vi "TestStand.DisplayError.vi"(8 "error in (no error)":errorcluster, 11 "Application Manager":refnum<k7>) -> (0 "error out":errorcluster)   [LabVIEW 2015, in "Main.GUI.lvlib"]
doc: "This VI displays an error dialog in the event of an error."
uses:
  Main.GUI.lvlib
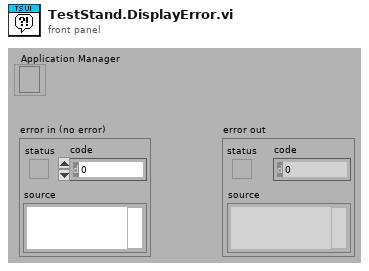
[diagram p1: front panel]
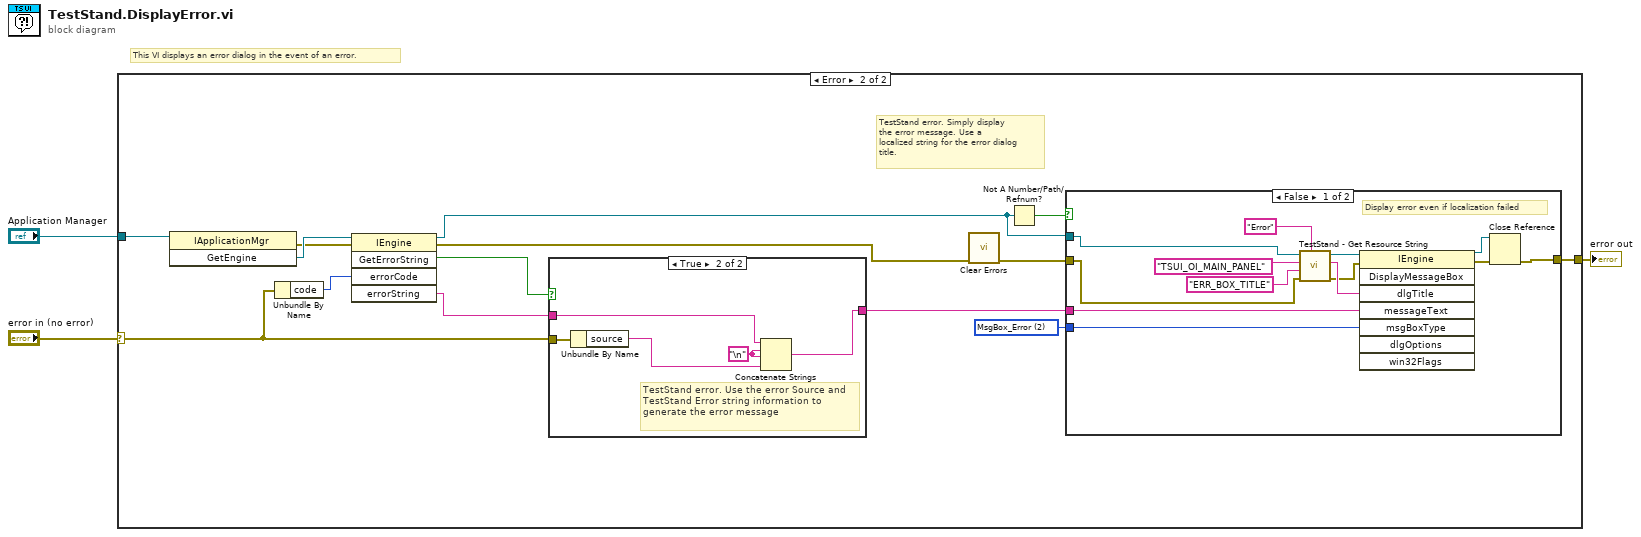
[diagram p0: block diagram]
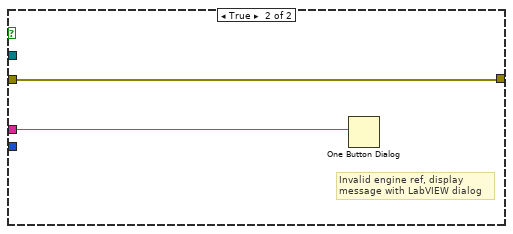
[diagram p3: hidden frame]
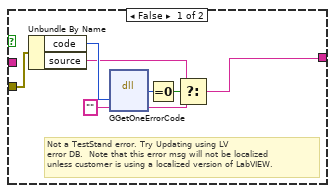
[diagram p4: hidden frame]
diagram:
  # "This VI displays an error dialog in the event of an error."
  n1 = case shown="Error" "error in (no error)" {
    selector: "error in (no error)" -> [w4 w16]
    tunnel: [w4 w12] -> w2
    tunnel: "Application Manager" -> [_ w13]
    frame No Error {
    }
    frame Error {
      w10 = 2 items=["MsgBox_Warning", "MsgBox_Information", "MsgBox_Error", "MsgBox_Custom"] ("msgBoxType")
      # "TestStand error. Simply display\nthe error message. Use a\nlocalized string for the error dialog\ntitle."
      n2 = invoke class="IApplicationMgr" method="GetEngine"(reference=w13) -> (error out=w14:errorcluster, "GetEngine"=w15:refnum<k7>)  [unwired: 2 in, 1 out]
      n3 = Unbundle By Name(w16) -> ("code"=w18:i32)
      n4 = invoke class="IEngine" method="GetErrorString"(reference=w15, error in=w14, "errorCode"=w18) -> (reference out=w5:refnum<k7>, error out=w6:errorcluster, "GetErrorString"=w17:bool, "errorString"=w8:string)  [unwired: 2 in, 1 out]
      n5 = case shown="True" w17 {
        tunnel: w16 -> [w35 w43]
        tunnel: [w34 w45] -> w11
        tunnel: w8 -> [_ w44]
        frame False {
          # "Not a TestStand error. Try Updating using LV\nerror DB.  Note that this error msg will not be localized\nunless customer is using a localized version of LabVIEW."
          n6 = Unbundle By Name(w35) -> ("code"=w37:i32, "source"=w36:string)
          n7 = dll-call lib="LabVIEW" fn="GGetOneErrorCode"("errorCode"=w37, "" ("input param")) -> (w40:u8, w38:string)  [unwired: 4 in, 2 out]
          n8 = Equal To 0?(x=w40) -> (x = 0?=w39:bool)
          n9 = Select(t=w36, s=w39, f=w38) -> (s? t:f=w34:string)
        }
        frame True {
          w46 = "\n"
          # "TestStand error. Use the error Source and TestStand Error string information to generate the error message"
          n10 = Unbundle By Name(w43) -> ("source"=w42:string)
          n11 = Concatenate Strings(w44, w46, w46, w42) -> (w45:string)
        }
      }
      n12 = call <vilib>:"Clear Errors.vi"("error in (no error)"=w6) -> ("error out"=w7:errorcluster)  [unwired: 1 in, 5 out]
      n13 = Not A Number/Path/Refnum?(number/path/refnum=w5) -> (NaN/Path/Refnum?=w9:bool)
      n14 = case shown="False" w9 {
        tunnel: [w31 w32] -> w12
        tunnel: w10 -> [w30 _]
        tunnel: w5 -> [w22 _]
        tunnel: w7 -> [w21 w32]
        tunnel: w11 -> [w27 w33]
        frame False {
          # "Display error even if localization failed"
          n15 = call <vilib>:"TestStand - Get Resource String.vi"("Default String"="Error", "error in (no error)"=w21, "Symbol"="ERR_BOX_TITLE", "Category"="TSUI_OI_MAIN_PANEL", "Engine Reference In"=w22) -> ("error out"=w19:errorcluster, "Resource String"=w24:string, "Engine Reference Out"=w20:refnum<k7>)  [unwired: 4 out]
          n16 = invoke class="IEngine" method="DisplayMessageBox"(reference=w20, error in=w19, "dlgTitle"=w24, "messageText"=w27, "msgBoxType"=w30) -> (reference out=w28:refnum<k7>, error out=w29:errorcluster)  [unwired: 3 in, 6 out]
          n17 = Close Reference(reference=w28, error in (no error)=w29) -> (error out=w31:errorcluster)
        }
        frame True {
          # "Invalid engine ref, display\nmessage with LabVIEW dialog"
          n18 = One Button Dialog(message=w33) -> ()  [unwired: 2 out]
        }
      }
    }
  }
  "error out" <- w2
